vi "Chamber controller Dec 14 2017.vi"() -> ()   [LabVIEW 2014]
doc: "This template is for the Queued Message Handler design pattern.\n\nThe Event Handling Loop generates messages based on user interface actions.\n\nThe Message Handling Loop processes messages generated by the Event Handling Loop, or by other messages. The messages are string values, so new messages can be added easily to the Message Cases case structure in the Message Handling Loop. Each message cluster can also provide an optional value for Message Data, which is a variant that can be converted to whatever message-specific data is required."
uses:
  <vilib>/Analysis/baseanly.llb/Mean (DBL).vi
  <vilib>/Instr/_visa.llb/VISA Configure Serial Port (Instr).vi
  Environmental Chamber LabVIEW and Instruments/Drivers and Software/Keithley 2100 Series/Public/Configure/Configure 2 Wire Resistance.vi
  <vilib>/Utility/file.llb/Write To Spreadsheet File (string).vi
  <vilib>/Utility/file.llb/Read From Spreadsheet File (string).vi
  Environmental Chamber LabVIEW and Instruments/Drivers and Software/LabVIEW 8.2 Drivers/keithley_24xx/Keithley 24XX/Public/Data/Read (Single Point).vi
  Environmental Chamber LabVIEW and Instruments/Drivers and Software/keithley_6430/Keithley 6430/Public/Data/Read (Single Point).vi
  Environmental Chamber LabVIEW and Instruments/Drivers and Software/keithley_6430/Keithley 6430/Keithley 6430.lvlib
  Environmental Chamber LabVIEW and Instruments/Drivers and Software/Keithley 2100 Series/Keithley 2100 Series.lvlib
  Environmental Chamber LabVIEW and Instruments/Drivers and Software/keithley_24xx/Keithley 24XX/Keithley 24XX.lvlib
  <vilib>/Analysis/NI_AALBase.lvlib
panel:
  in  "K2420 Applied Voltage (V)":dbl=0.05
  in  "SYSTEM CONTROL":T1={"valve % open"=0.0, "Desired pressure"=0.0, "set Vapor sccm"=0.0, "set Gas sccm"=0.0, "Valve mode"=enum."% Open", "Pressure Mode"=enum."Abs. pressure", "analyte partial pressure"=23.8, "Actual"=0.0, "Read pressure (Torr)"=0.0, "Read vapor flow (sccm)"=0.0, "Read gas flow (sccm)"=0.0, "Save now"=FALSE, "Stop after seq."=TRUE, "Turbo pump\nauto on"=TRUE, "Integrate points"=0} caption="Pressure settings" {"Integrate points" min=0 max=100 step=1; "analyte partial pressure" min=0.0 max=100.0 step=5.0; "set Gas sccm" min=0 max=200 step=5; "set Vapor sccm" min=0 max=200 step=5; "Desired pressure" min=0.0 max=760.0 step=5.0; "valve % open" min=0.0 max=100.0 step=5.0 format="%#_2f"}
  in  "SAVE SAMPLE / ANALYTE NAMES":T2={"QCM1"="", "QCM2"="", "QCM3"="", "QCM4"="broken", "QCM5"="NOT WORKING", "QCM6"="", "SRS"="bareAu", "K-2420"="", "K-6430"="", "K-2100"="", "Gas"="NOT WORKING", "Vapor"="H2O", "Notes"=""} caption="Save samplffe names"
  in  "Clear all charts":bool
  out "K-6430":dbl(graph)
  out "K-2420":dbl(graph)
  out "File":path caption="DATA FILE"
  in  "Stop":bool
  out "QCM plot":T3(graph)
  out "K-2100":dbl(graph)
  out "State date/time":string caption="Program start time"
  out "J-KEM temp":dbl(graph)
  out "saving data?":bool
  out "pressure chart":dbl(graph)
  out "arduino qcm stack plot":T4(graph)
  in  "SEQUENCE":T5 {"preview" items=["pressure", "gas flow", "vapor flow", "bias"]}
  # "100"
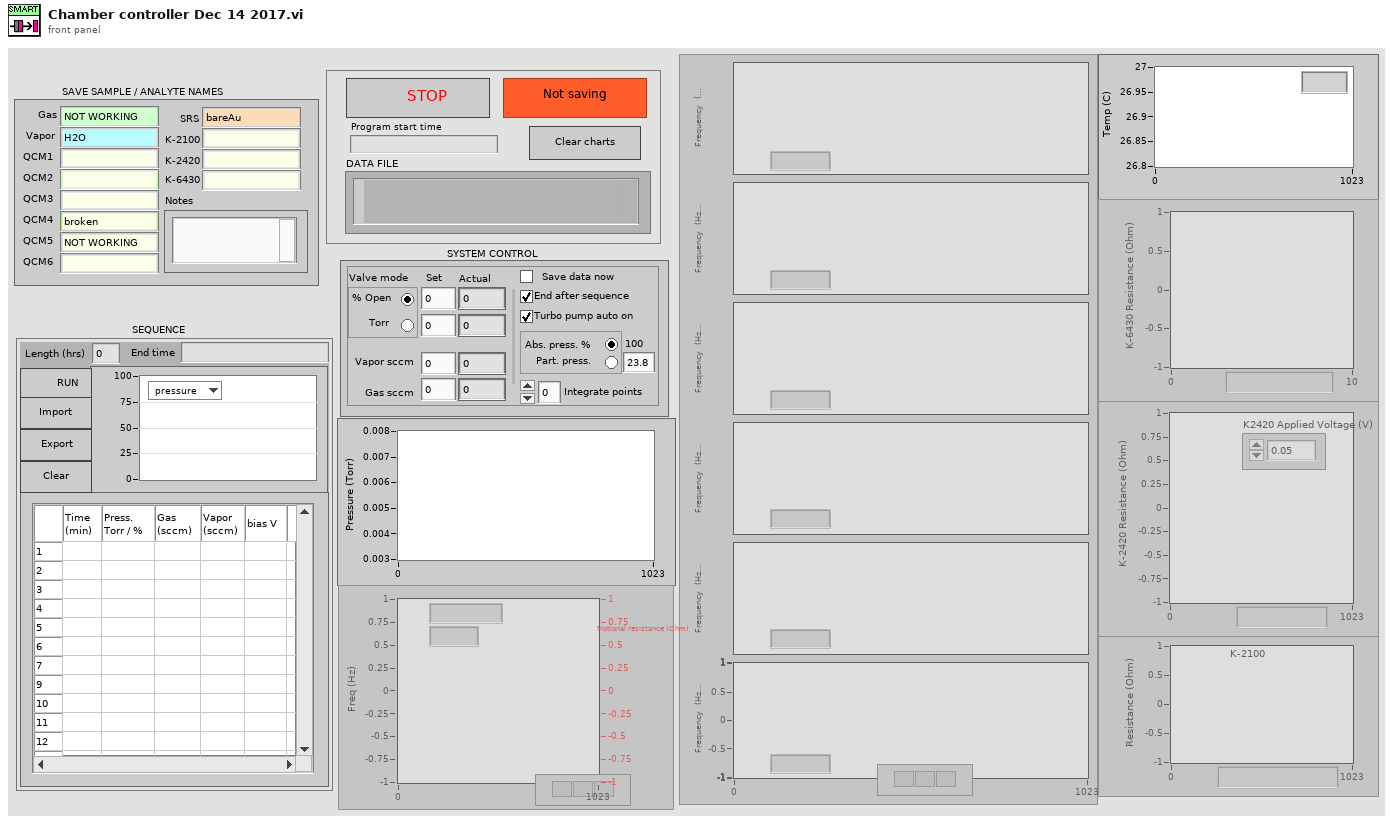
[diagram p1: front panel]
types:
  T1 = cluster{"valve % open":dbl, "Desired pressure":dbl, "set Vapor sccm":sgl, "set Gas sccm":sgl, "Valve mode":enum32{"% Open", "Torr "}, "Pressure Mode":enum32{"Abs. pressure", " Part. pressure"}, "analyte partial pressure":dbl, "Actual":dbl, "Read pressure (Torr)":dbl, "Read vapor flow (sccm)":dbl, "Read gas flow (sccm)":dbl, "Save now":bool, "Stop after seq.":bool, "Turbo pump\nauto on":bool, "Integrate points":i32}
  T2 = cluster{"QCM1":string, "QCM2":string, "QCM3":string, "QCM4":string, "QCM5":string, "QCM6":string, "SRS":string, "K-2420":string, "K-6430":string, "K-2100":string, "Gas":string, "Vapor":string, "Notes":string}
  T3 = cluster{"Frequency out":dbl, "Resistance out":dbl}
  T4 = cluster{"[0]":dbl, "[1]":dbl, "[2]":dbl, "[3]":dbl, "[4]":dbl, "[5]":dbl}
  T5 = cluster{"Run Sequence":bool, "User-defined\nsequence":string[][], "preview":u16, "Sequence\npreview":cluster{dbl[], dbl[]}[], "Save sequence":bool, "Clear sequence":bool, "Import sequence file":bool, "Length (hrs)":dbl, "End time":string}
  T6 = cluster{"Keithley 6430":bool, "J-KEM":bool, "Keithley 2420":bool, "Keithley 2100":bool, "SRS QCM":bool, "Pressure control":bool, "Arduino":bool}
  T7 = cluster{"Arduino 1":refnum<visa-resource-name>, "Arduino 2":refnum<visa-resource-name>, "Arduino 3":refnum<visa-resource-name>, "Arduino 4":refnum<visa-resource-name>, "Arduino 5":refnum<visa-resource-name>, "Arduino 6":refnum<visa-resource-name>}
  T8 = enum8{"Enabled", "Disabled", "Disabled and Grayed Out"}
  T9 = enum16{"open", "open or create", "create or replace", "create", "open (read only)"}
  T10 = cluster{"[0]":dbl, "[1]":dbl, "[2]":dbl, "[3]":dbl, "[4]":dbl, "[5]":dbl}[]
  T11 = cluster{"Frequency out":dbl, "Resistance out":dbl}[]
  T12 = cluster{"VISA resource name":refnum<visa-resource-name>, "error out":errorcluster, bool}
  T13 = cluster{"VISA resource name out":refnum<visa-resource-name>, "error out":errorcluster, bool}
  T14 = cluster{bool, "task out":refnum<k21>, "error out":errorcluster, "task out":refnum<k21>, "error out":errorcluster, "turbo pump":refnum<visa-resource-name>, "error out":errorcluster}
  T15 = cluster{bool, "task out":refnum<k21>, "error out":errorcluster, "task out":refnum<k21>, "error out":errorcluster, "VISA resource name out":refnum<visa-resource-name>, "error out":errorcluster}
  T16 = cluster{bool, "VISA resource name":refnum<visa-resource-name>, "error out":errorcluster}
  T17 = cluster{bool, "VISA resource name out":refnum<visa-resource-name>, "error out":errorcluster}
  T18 = cluster{bool, "VISA in":refnum<visa-resource-name>, "error out":errorcluster}
  T19 = cluster{bool, "VISA out":refnum<visa-resource-name>, "error out":errorcluster}
  T20 = cluster{"Arduino address":refnum<visa-resource-name>, "error in (no error)":errorcluster, "Arduino address 2":refnum<visa-resource-name>, "error in (no error) 2":errorcluster, "Arduino address 3":refnum<visa-resource-name>, "error in (no error) 3":errorcluster, "Arduino address 4":refnum<visa-resource-name>, "error in (no error) 4":errorcluster, "Arduino address 5":refnum<visa-resource-name>, "error in (no error) 5":errorcluster, "Arduino address 6":refnum<visa-resource-name>, "error in (no error) 6":errorcluster, "arduinos on?":bool}
  T21 = cluster{"valve % open":dbl, "Desired pressure":dbl, "set Vapor sccm":sgl, "set Gas sccm":sgl, "Valve mode":enum32{"% Open", "Torr "}, "Pressure Mode":enum32{"Abs. pressure", " Part. pressure"}, "analyte partial pressure":dbl}
  T22 = cluster{"Boolean":bool, "VISA resource name out":refnum<visa-resource-name>, "error out":errorcluster}
  T23 = cluster{"Boolean":bool, "VISA out":refnum<visa-resource-name>, "error out":errorcluster}
  T24 = cluster{"Boolean":bool, "Arduino address":refnum<visa-resource-name>, "error in (no error)":errorcluster, "Arduino address 2":refnum<visa-resource-name>, "error in (no error) 2":errorcluster, "Arduino address 3":refnum<visa-resource-name>, "error in (no error) 3":errorcluster, "Arduino address 4":refnum<visa-resource-name>, "error in (no error) 4":errorcluster, "Arduino address 5":refnum<visa-resource-name>, "error in (no error) 5":errorcluster, "Arduino address 6":refnum<visa-resource-name>, "error in (no error) 6":errorcluster}
  T25 = cluster{"arduino addresses out":cluster{"Boolean":bool, "Arduino address":refnum<visa-resource-name>, "error in (no error)":errorcluster, "Arduino address 2":refnum<visa-resource-name>, "error in (no error) 2":errorcluster, "Arduino address 3":refnum<visa-resource-name>, "error in (no error) 3":errorcluster, "Arduino address 4":refnum<visa-resource-name>, "error in (no error) 4":errorcluster, "Arduino address 5":refnum<visa-resource-name>, "error in (no error) 5":errorcluster, "Arduino address 6":refnum<visa-resource-name>, "error in (no error) 6":errorcluster}, cluster{bool, "VISA resource name out":refnum<visa-resource-name>, "error out":errorcluster}, "Address out":cluster{"Boolean":bool, "VISA resource name out":refnum<visa-resource-name>, "error out":errorcluster}, cluster{bool, "VISA resource name out":refnum<visa-resource-name>, "error out":errorcluster}, cluster{bool, "VISA resource name out":refnum<visa-resource-name>, "error out":errorcluster}, "SRS address out":cluster{"Boolean":bool, "VISA out":refnum<visa-resource-name>, "error out":errorcluster}}
  T26 = cluster{"User-defined\nsequence":string[][], "Present (s)":dbl, "current  step # in":i32, "sequence end time in":timestamp}
  T27 = cluster{"current  step # in":i32, "sequence end time in":timestamp, "Boolean":bool}
  T28 = cluster{"press/RH/gas/vapor":cluster{"pressure":string, "RH":string, "gas flow":string, "vapor flow":string}, "Cluster":cluster{"Valve position (%)":dbl, "read pressure":dbl, "read vapor flow":dbl, "read gas flow":dbl}}
  T29 = cluster{"Boolean":bool, "task out":refnum<k21>, "error out":errorcluster, "task out":refnum<k21>, "error out":errorcluster, "VISA resource name out":refnum<visa-resource-name>, "error out":errorcluster}
  T30 = cluster{"pressure":string, "RH":string, "gas flow":string, "vapor flow":string}
  T31 = cluster{"Valve position (%)":dbl, "read pressure":dbl, "read vapor flow":dbl, "read gas flow":dbl}
  T32 = cluster{"[0]":string, "[1]":string, "[2]":string, "[3]":string, "[4]":string, "[5]":string}
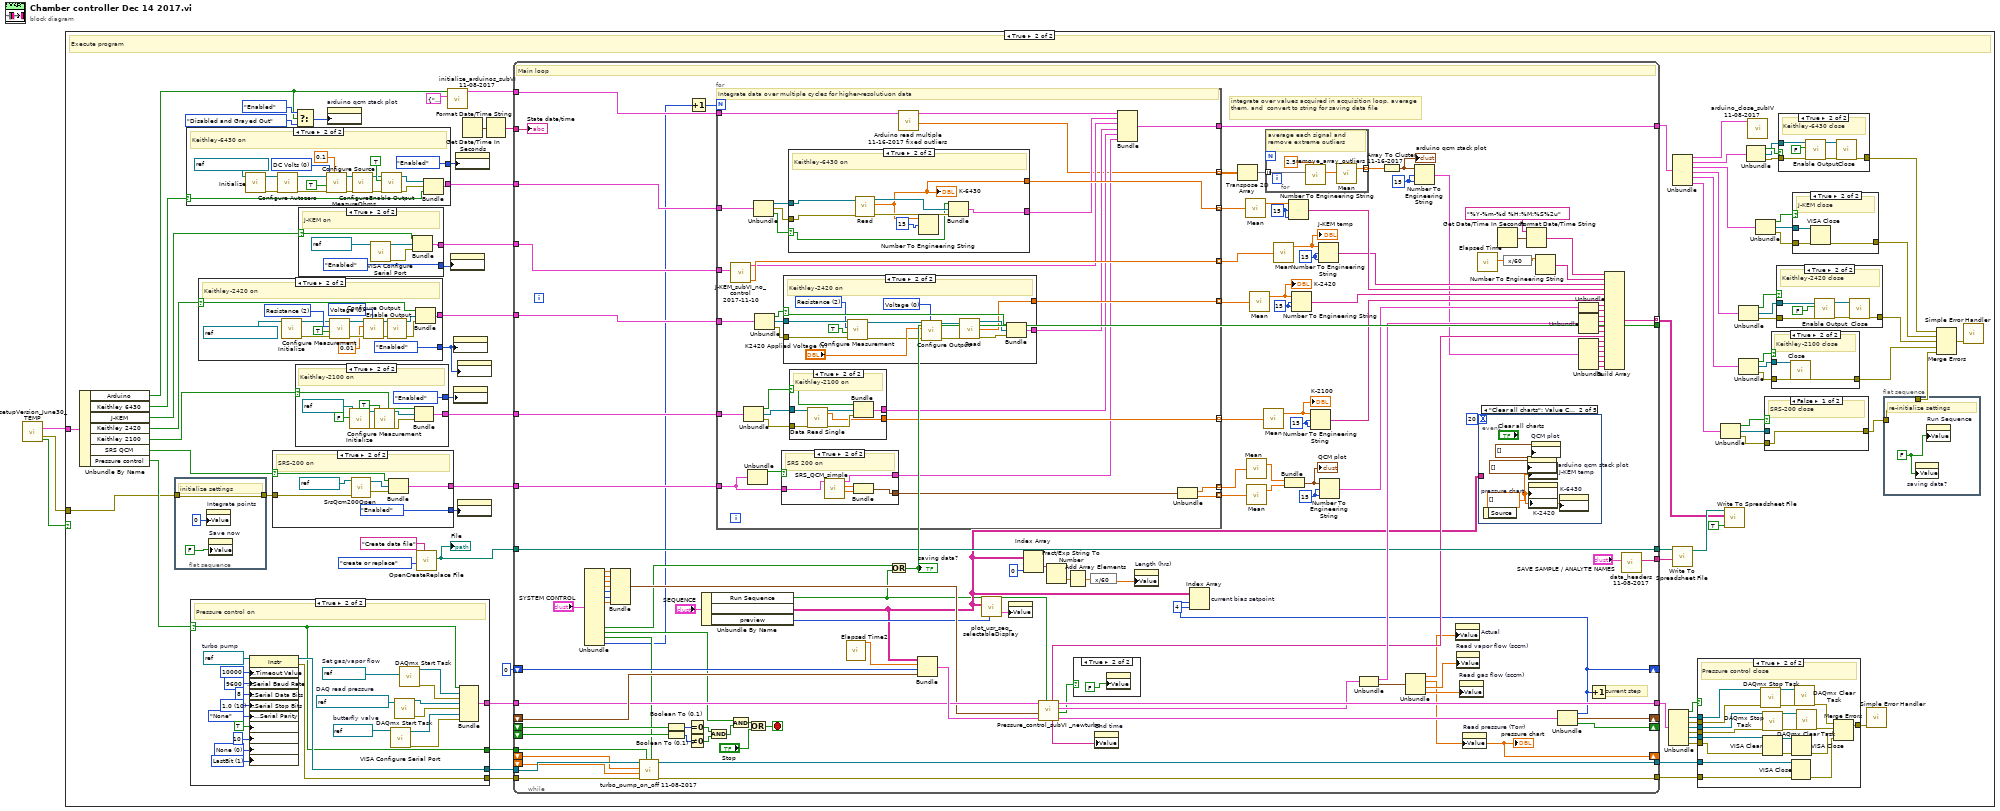
[diagram p0: block diagram]
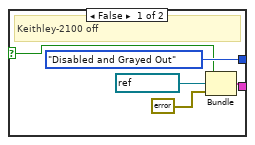
[diagram p4: hidden frame]
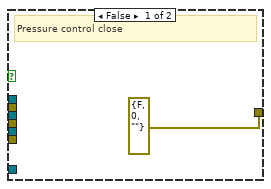
[diagram p5: hidden frame]
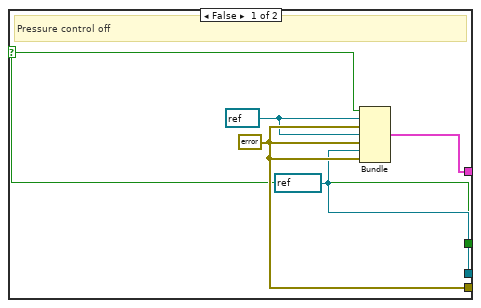
[diagram p6: hidden frame]
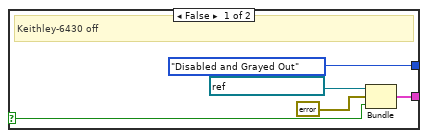
[diagram p8: hidden frame]
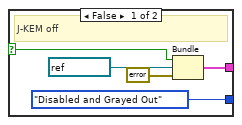
[diagram p10: hidden frame]
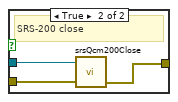
[diagram p11: hidden frame]
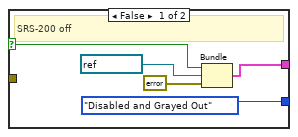
[diagram p12: hidden frame]
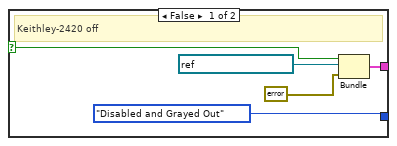
[diagram p14: hidden frame]
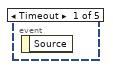
[diagram p15: hidden frame]
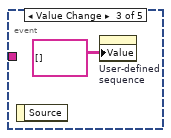
[diagram p16: hidden frame]
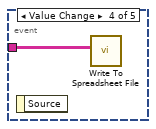
[diagram p17: hidden frame]
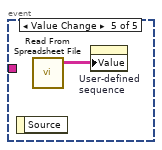
[diagram p18: hidden frame]
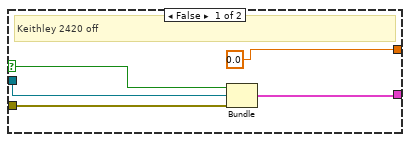
[diagram p19: hidden frame]
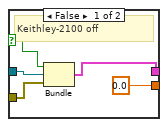
[diagram p20: hidden frame]
diagram:
  n1 = call "setupVersion_June30_TEMP.vi"() -> ("Instruments on/off"=w1:T6, "error IO"=w2:errorcluster, "OK"=w3:bool)  [unwired: 13 in]
  n2 = case shown="True" w3 {
    tunnel: w2 -> [_ w41]
    tunnel: w1 -> [_ w48]
    frame False {
      # "Cancel program"
    }
    frame True {
      # "Execute program"
      n3 = Unbundle By Name(w48) -> ("Arduino"=w19:bool, "Keithley 6430"=w47:bool, "J-KEM"=w46:bool, "Keithley 2420"=w45:bool, "Keithley 2100"=w44:bool, "SRS QCM"=w43:bool, "Pressure control"=w42:bool)
      n4 = flat-sequence {
        tunnel: [w86] -> w40
        tunnel: w41 -> [w86]
        frame #0 {
          # "initialize settings"
          n5 = property on="Integrate points" class="DigNum (strict)"("Value"=0) -> ()  [unwired: 2 in, 2 out]
          n6 = property on="Save now" class="Bool (strict)"("Value"=FALSE) -> ()  [unwired: 2 in, 2 out]
        }
      }
      n7 = case shown="True" w47 {
        selector: w47 -> [w164 w184]
        tunnel: [T8."Disabled and Grayed Out" ("Disabled") T8."Enabled" ("Disabled")] -> w26
        tunnel: [w163 w183] -> w24
        frame False {
          # "Keithley-6430 off"
          n8 = Bundle("VISA resource name"=refnum<visa-resource-name> "GPIB0::29::INSTR", "error out"=errorcluster {"status"=FALSE, "code"=0, "source"=""}, w164) -> (w163:T12)  [unwired: 1 in]
        }
        frame True {
          w171 = u16 0 items=["DC Volts", "DC Current"] ("Source Function (0: DC Volts)")
          # "Keithley-6430 on"
          n9 = call "Initialize.vi"("VISA resource name"=refnum<visa-resource-name> "GPIB2::19::INSTR") -> ("error out"=w177:errorcluster, "VISA resource name out"=w178:refnum<visa-resource-name>)  [unwired: 4 in, 5 out]
          n10 = call "Configure Autozero.vi"("error in (no error)"=w177, "VISA resource name"=w178) -> ("error out"=w174:errorcluster, "VISA resource name out"=w176:refnum<visa-resource-name>)  [unwired: 8 in]
          n11 = call "Configure Source.vi"("V-Source Level [V]"=0.1, "error in (no error)"=w174, "Auto Range (T:Enable)"=TRUE, "Source Function (0: DC Volts)"=w171, "VISA resource name"=w176) -> ("error out"=w173:errorcluster, "VISA resource name out"=w175:refnum<visa-resource-name>)  [unwired: 5 in]
          n12 = call "Configure MeasureOhms.vi"("error in (no error)"=w173, "VISA resource name"=w175) -> ("error out"=w182:errorcluster, "VISA resource name out"=w180:refnum<visa-resource-name>)  [unwired: 4 in, 4 out]
          n13 = call "Enable Output.vi"("error in (no error)"=w182, "Enable Output (F:Off)"=TRUE ("Output (F:Off)"), "VISA resource name"=w180) -> ("error out"=w169:errorcluster, "VISA resource name out"=w170:refnum<visa-resource-name>)  [unwired: 7 out]
          n14 = Bundle("VISA resource name out"=w170, "error out"=w169, w184) -> (w183:T13)  [unwired: 1 in]
        }
      }
      n15 = case shown="True" w42 {
        selector: w42 -> [w128 w134]
        tunnel: [w132 w135] -> w39
        tunnel: [w131 w133] -> w31
        tunnel: [w129 w136] -> w32
        tunnel: [w128 w134] -> w30
        frame False {
          w129 = refnum<visa-resource-name> refnum ("turbo pump")
          w130 = refnum<k21> refnum ("task out")
          w131 = errorcluster {"status"=FALSE, "code"=0, "source"=""} ("error out")
          # "Pressure control off"
          n16 = Bundle(w128, "task out"=w130, "error out"=w131, "task out"=w130, "error out"=w131, "turbo pump"=w129, "error out"=w131) -> (w132:T14)  [unwired: 1 in]
        }
        frame True {
          w140 = u16 1 items=["None", "LastBit", "TermChar"] ("Serial Settings:Serial End Mode for Reads")
          w138 = u16 0 items=["None", "XON/XOFF", "RTS/CTS", "XON/XOFF & RTS/CTS", "DTR/DSR", "XON/XOFF & DTR/DSR"] ("flow control (0:none)")
          w141 = u16 10 items=["1.0"=10, "1.5"=15, "2.0"=20] ("stop bits (10: 1 bit)")
          w137 = refnum<visa-resource-name> "COM7"  # turbo pump
          w153 = refnum<visa-resource-name> "COM5"  # butterfly valve
          w154 = refnum<k21> "Setflow"  # Set gas/vapor flow
          w155 = refnum<k21> "AllDaqReadings"  # DAQ read pressure
          # "Pressure control on"
          n17 = property class="Instr"(reference=w137, "General Settings:Timeout Value"=u32 10000 ("timeout (10sec)"), "Serial Settings:Serial Baud Rate"=u32 9600 ("baud rate (9600)"), "Serial Settings:Serial Data Bits"=u16 8 ("data bits (8)"), "Serial Settings:Serial Stop Bits"=w141, "Serial Settings:Serial Parity"=enum16{"None", "Odd", "Even", "Mark", "Space"}."None" ("parity (0:none)"), "Message Based Settings:Termination Character Enable"=TRUE ("Enable Termination\nChar (T)"), "Message Based Settings:Termination Character"=u8 10 ("termination char\n(0xA = '\\n' = LF)"), "Serial Settings:Serial Flow Control"=w138, "Serial Settings:Serial End Mode for Reads"=w140) -> (reference out=w136:refnum<visa-resource-name>, error out=w133:errorcluster)  [unwired: 1 in]
          n18 = call-poly "VISA Configure Serial Port"("VISA resource name"=w153) -> ("VISA resource name out"=w148:refnum<visa-resource-name>, "error out"=w147:errorcluster)  [unwired: 13 in]
          n19 = call <vilib>:"DAQmx Start Task.vi"("task/channels in"=w155) -> ("task out"=w150:refnum<k21>, "error out"=w149:errorcluster)  [unwired: 13 in]
          n20 = call <vilib>:"DAQmx Start Task.vi"("task/channels in"=w154) -> ("task out"=w152:refnum<k21>, "error out"=w151:errorcluster)  [unwired: 13 in]
          n21 = Bundle(w134, "task out"=w152, "error out"=w151, "task out"=w150, "error out"=w149, "VISA resource name out"=w148, "error out"=w147) -> (w135:T15)  [unwired: 1 in]
        }
      }
      n22 = case shown="True" w45 {
        selector: w45 -> [w227 w232]
        tunnel: [T8."Disabled and Grayed Out" ("Disabled") T8."Enabled" ("Disabled")] -> w4
        tunnel: [w225 w229] -> w23
        frame False {
          # "Keithley-2420 off"
          n23 = Bundle(w227, "VISA resource name"=refnum<visa-resource-name> "GPIB1::24::INSTR", "error out"=errorcluster {"status"=FALSE, "code"=0, "source"=""}) -> (w225:T16)  [unwired: 1 in]
        }
        frame True {
          w238 = u16 0 items=["Voltage", "Current"] ("Source Mode  (0: Voltage)")
          w243 = u16 2 items=["Volts", "Current", "Resistance"] ("Function (0: Volts)")
          # "Keithley-2420 on"
          n24 = call "Initialize.vi"("VISA resource name"=refnum<visa-resource-name> "GPIB1::24::INSTR") -> ("error out"=w233:errorcluster, "VISA resource name out"=w234:refnum<visa-resource-name>)  [unwired: 9 in]
          n25 = call "Configure Measurement.vi"("error in (no error)"=w233, "Enable Auto Range (T:Enable)"=TRUE, "Function (0: Volts)"=w243, "VISA resource name"=w234) -> ("error out"=w242:errorcluster, "VISA resource name out"=w241:refnum<visa-resource-name>)  [unwired: 6 in]
          n26 = call "Configure Output.vi"("Source Mode  (0: Voltage)"=w238, "error in (no error)"=w242, "Output Level (0)"=0.01 ("K2420 Applied Voltage (V) 2"), "VISA resource name"=w241) -> ("error out"=w240:errorcluster, "VISA resource name out"=w239:refnum<visa-resource-name>)  [unwired: 6 in]
          n27 = call "Enable Output.vi"("error in (no error)"=w240, "VISA resource name"=w239) -> ("error out"=w230:errorcluster, "VISA resource name out"=w231:refnum<visa-resource-name>)  [unwired: 8 in]
          n28 = Bundle(w232, "VISA resource name out"=w231, "error out"=w230) -> (w229:T17)  [unwired: 1 in]
        }
      }
      n29 = case shown="True" w43 {
        selector: w43 -> [w206 w212]
        tunnel: w40 -> [_ w215]
        tunnel: [T8."Disabled and Grayed Out" ("Disabled") T8."Enabled" ("Disabled")] -> w63
        tunnel: [w205 w211] -> w21
        frame False {
          # "SRS-200 off"
          n30 = Bundle(w206, "VISA in"=refnum<visa-resource-name> "COM6", "error out"=errorcluster {"status"=FALSE, "code"=0, "source"=""}) -> (w205:T18)  [unwired: 1 in]
        }
        frame True {
          # "SRS-200 on"
          n31 = call "SrsQcm200Open.vi"("error in"=w215, "VISA in"=refnum<visa-resource-name> "COM6") -> ("error out"=w210:errorcluster, "VISA out"=w213:refnum<visa-resource-name>)  [unwired: 3 in]
          n32 = Bundle(w212, "VISA out"=w213, "error out"=w210) -> (w211:T19)  [unwired: 1 in]
        }
      }
      n33 = Select(t=T8."Enabled" ("Disabled"), s=w19, f=T8."Disabled and Grayed Out" ("Disabled")) -> (s? t:f=w27:T8)
      n34 = case shown="True" w44 {
        selector: w44 -> [w96 w100]
        tunnel: [T8."Disabled and Grayed Out" ("Disabled") T8."Enabled" ("Disabled")] -> w58
        tunnel: [w93 w101] -> w22
        frame False {
          # "Keithley-2100 off"
          n35 = Bundle(w96, "VISA resource name out"=refnum<visa-resource-name> "K-2100", "error out"=errorcluster {"status"=FALSE, "code"=0, "source"=""}) -> (w93:T17)  [unwired: 1 in]
        }
        frame True {
          # "Keithley-2100 on"
          n36 = call "Initialize.vi"("VISA resource name"=refnum<visa-resource-name> "K-2100", "Reset? (T: Reset)"=FALSE) -> ("VISA resource name out"=w105:refnum<visa-resource-name>, "error out"=w104:errorcluster)  [unwired: 16 in]
          n37 = call-poly "Configure Measurement.vi"("VISA resource name"=w105, "error in (no error)"=w104, "Auto Range? (T: Auto)"=TRUE) -> ("VISA resource name out"=w99:refnum<visa-resource-name>, "error out"=w98:errorcluster)  [unwired: 15 in]
          n38 = Bundle(w100, "VISA resource name out"=w99, "error out"=w98) -> (w101:T17)  [unwired: 1 in]
        }
      }
      n39 = case shown="True" w46 {
        selector: w46 -> [w191 w197]
        tunnel: [w192 w198] -> w76
        tunnel: [T8."Disabled and Grayed Out" ("Disabled") T8."Enabled" ("Disabled")] -> w25
        frame False {
          # "J-KEM off"
          n40 = Bundle(w191, "VISA resource name"=refnum<visa-resource-name> "COM3", "error out"=errorcluster {"status"=FALSE, "code"=0, "source"=""}) -> (w192:T16)  [unwired: 1 in]
        }
        frame True {
          # "J-KEM on"
          n41 = call-poly "VISA Configure Serial Port"("VISA resource name"=refnum<visa-resource-name> "COM3") -> ("VISA resource name out"=w199:refnum<visa-resource-name>, "error out"=w196:errorcluster)  [unwired: 13 in]
          n42 = Bundle(w197, "VISA resource name out"=w199, "error out"=w196) -> (w198:T17)  [unwired: 1 in]
        }
      }
      n43 = property on="arduino qcm stack plot" class="WFChart (strict)"("DisabledEnum"=w27) -> ()  [unwired: 2 in, 2 out]
      n44 = call "OpenCreateReplace File.vi"("prompt"="Create data file", "function (open:0)"=T9."create or replace") -> ("new file path"=w20:path)  [unwired: 6 in, 3 out]
      "File" <- w20
      n45 = call "initialize_arduinos_subVI 11-08-2017.vi"("arduino 1-6 addresses"=T7 {"Arduino 1"="COM25", "Arduino 2"="COM48", "Arduino 3"="COM21", "Arduino 4"="COM22", "Arduino 5"="COM23", "Arduino 6"="COM24"} ("Arduino COMs"), "arduinos on?"=w19) -> ("arduino addresses out"=w61:T20)  [unwired: 9 in]
      n46 = property on="J-KEM temp" class="WFChart (strict)"("DisabledEnum"=w25) -> ()  [unwired: 2 in, 2 out]
      n47 = property on="K-2420" class="WFChart (strict)"("DisabledEnum"=w4) -> ()  [unwired: 2 in, 2 out]
      n48 = property on="K-2100" class="WFChart (strict)"("DisabledEnum"=w58) -> ()  [unwired: 2 in, 2 out]
      n49 = property on="K-6430" class="WFChart (strict)"("DisabledEnum"=w26) -> ()  [unwired: 2 in, 2 out]
      n50 = property on="K2420 Applied Voltage (V)" class="DigNum (strict)"("DisabledEnum"=w4) -> ()  [unwired: 2 in, 2 out]
      n51 = property on="QCM plot" class="WFChart (strict)"("DisabledEnum"=w63) -> ()  [unwired: 2 in, 2 out]
      n52 = Get Date/Time In Seconds() -> (seconds since 1Jan1904=w5:timestamp)
      n53 = Format Date/Time String(seconds (now)=w5) -> (date/time string=w57:string)  [unwired: 2 in]
      n54 = while {
        tunnel: [w364] -> w62 mode=indexing if=w351
        tunnel: w76 -> [w366]
        tunnel: [w334] -> w68
        tunnel: w20 -> [w334]
        tunnel: [w351] -> _
        tunnel: w61 -> [w311]
        tunnel: [w323] -> w60
        tunnel: w57 -> [w346]
        tunnel: w39 -> [w332]
        shift-right: [w307] -> _
        shift-left: 0 ("1st step") -> [w338]
        shift-right: [w343] -> _
        shift-left: _ -> [w341]
        shift-right: [w342] -> _
        shift-left: _ -> [w340]
        shift-left: _ -> [w339]
        tunnel: [w337] -> w53
        tunnel: w32 -> [w331]
        tunnel: w31 -> [w330]
        tunnel: w30 -> [w310]
        tunnel: [w328] -> w29
        tunnel: [w329] -> w28
        tunnel: w24 -> [w316]
        tunnel: w23 -> [w315]
        tunnel: w22 -> [w314]
        tunnel: w21 -> [w313]
        shift-right: [w246] -> _
        shift-left: _ -> [w309]
        shift-left: _ -> [w308]
        tunnel: [w281] -> w12
        stop <- w353 stop-if-true
        w273 = i16 15 ("width (-)")
        w274 = i16 15 ("width (-)")
        w275 = i16 15 ("width (-)")
        w276 = i16 15 ("width (-)")
        w277 = i16 15 ("width (-)")
        w278 = i16 15 ("width (-)")
        # "current step"
        # "integrate over values acquired in acquisition loop, average them, and  convert to string for saving data file"
        # "Main loop"
        n55 = Unbundle("SYSTEM CONTROL") -> ("valve % open"=w266:dbl, "Desired pressure"=w265:dbl, "set Vapor sccm"=w264:sgl, "set Gas sccm"=w263:sgl, "Valve mode"=w262:enum32{"% Open", "Torr "}, "Pressure Mode"=w261:enum32{"Abs. pressure", " Part. pressure"}, "analyte partial pressure"=w260:dbl, "Save now"=w251:bool, "Stop after seq."=w250:bool, "Turbo pump\nauto on"=w249:bool, "Integrate points"=w248:i32)  [unwired: 4 out]
        n56 = Bundle("valve % open"=w266, "Desired pressure"=w265, "set Vapor sccm"=w264, "set Gas sccm"=w263, "Valve mode"=w262, "Pressure Mode"=w261, "analyte partial pressure"=w260) -> (w267:T21)  [unwired: 1 in]
        n57 = call "turbo_pump_on_off 11-08-2017.vi"("Turbo pump\nauto on"=w249, "pressure control on?"=w310, "error in (no error)"=w330, "read pressure"=w308, "read pressure 2"=w309, "VISA Refnum in"=w331) -> ("error out"=w329:errorcluster, "VISA Refnum out"=w328:refnum<visa-resource-name>)  [unwired: 4 in]
        n58 = Boolean To (0,1)(Boolean=w340) -> (0, 1=w357:i16)
        n59 = Boolean To (0,1)(Boolean=w339) -> (0, 1=w356:i16)
        n60 = Equal To 0?(x=w357) -> (x = 0?=w354:bool)
        n61 = Not Equal To 0?(x=w356) -> (x != 0?=w355:bool)
        n62 = Increment(x=w248) -> (x+1=w280:i32)
        n63 = Unbundle By Name("SEQUENCE") -> ("Run Sequence"=w253:bool, "User-defined\nsequence"=w257:string[][], "preview"=w258:u16)
        n64 = And(x=w354, y=w355) -> (x .and. y?=w352:bool)
        n65 = for {
          N: w280 -> [_]
          tunnel: w316 -> [w407]
          tunnel: w315 -> [w404]
          tunnel: w314 -> [w400]
          tunnel: w313 -> [w381]
          tunnel: w311 -> [w380]
          tunnel: w366 -> [w408]
          tunnel: [w395] -> w302 mode=indexing
          tunnel: [w394] -> w296 mode=indexing
          tunnel: [w393] -> w299 mode=indexing
          tunnel: [w392] -> w294 mode=indexing
          tunnel: [w390] -> w292 mode=indexing
          tunnel: [w389] -> w291 mode=indexing
          tunnel: [w379] -> w286 mode=indexing
          tunnel: [w383] -> w281
          # "Integrate data over multiple cycles for higher-resolutiuon data"
          n66 = call "J-KEM_subVI_no_control 2017-11-10.vi"("Address in"=w408) -> ("Temp (C)"=w393:dbl, "Address out"=w387:T22)  [unwired: 9 in]
          n67 = Unbundle(w400) -> (w399:bool, "VISA resource name out"=w398:refnum<visa-resource-name>, "error out"=w397:errorcluster)
          n68 = Unbundle(w381) -> (w382:bool)  [unwired: 2 out]
          n69 = Unbundle(w407) -> ("VISA resource name out"=w406:refnum<visa-resource-name>, "error out"=w396:errorcluster, w405:bool)
          n70 = Unbundle(w404) -> (w403:bool, "VISA resource name out"=w402:refnum<visa-resource-name>, "error out"=w401:errorcluster)
          n71 = case "SRS QCM" shown="True" w382 {
            tunnel: [w454 w460] -> w384
            tunnel: [T3 {"Frequency out"=0.0, "Resistance out"=0.0} ("freq, MR") w457] -> w391
            tunnel: w381 -> [w454 w456]
            frame False {
              # "SRS QCM off"
            }
            frame True {
              # "SRS 200 on"
              n72 = call "SRS_QCM_simple.vi"("SRS address in"=w456) -> ("Resistance out"=w459:dbl, "Frequency out"=w458:dbl, "SRS address out"=w460:T23)  [unwired: 8 in]
              n73 = Bundle("Frequency out"=w458, "Resistance out"=w459) -> (w457:T3)  [unwired: 1 in]
            }
          }
          n74 = case shown="True" w403 {
            selector: w403 -> [w413 w428]
            tunnel: [w410 w427] -> w386
            tunnel: w402 -> [w412 w420]
            tunnel: w401 -> [w411 w418]
            tunnel: [sgl 0.0 ("Resistance") w415] -> w394
            frame False {
              # "Keithley 2420 off"
              n75 = Bundle(w413, "VISA resource name out"=w412, "error out"=w411) -> (w410:T17)  [unwired: 1 in]
            }
            frame True {
              w416 = u16 2 items=["Volts", "Current", "Resistance"] ("Function (0: Volts)")
              w424 = u16 0 items=["Voltage", "Current"] ("Source Mode  (0: Voltage)")
              # "Keithley-2420 on"
              n76 = call "Configure Measurement.vi"("error in (no error)"=w418, "Enable Auto Range (T:Enable)"=TRUE, "Function (0: Volts)"=w416, "VISA resource name"=w420) -> ("error out"=w417:errorcluster, "VISA resource name out"=w419:refnum<visa-resource-name>)  [unwired: 6 in]
              n77 = call "Configure Output.vi"("Source Mode  (0: Voltage)"=w424, "error in (no error)"=w417, "Output Level (0)"="K2420 Applied Voltage (V)", "VISA resource name"=w419) -> ("error out"=w422:errorcluster, "VISA resource name out"=w423:refnum<visa-resource-name>)  [unwired: 6 in]
              n78 = call-poly "Read.vi"("VISA resource name"=w423, "error in (no error)"=w422) -> ("VISA resource name out"=w426:refnum<visa-resource-name>, "Resistance"=w415:sgl, "error out"=w425:errorcluster)  [unwired: 7 in, 4 out]
              n79 = Bundle(w428, "VISA resource name out"=w426, "error out"=w425) -> (w427:T17)  [unwired: 1 in]
            }
          }
          n80 = case "Keithley 6430" shown="True" w405 {
            selector: w405 -> [w445 w448]
            tunnel: w406 -> [w444 w450]
            tunnel: [w443 w447] -> w388
            tunnel: w396 -> [w442 w449]
            tunnel: [0.0 ("K6340 Bias (V)") w446] -> w395
            frame False {
              # "Keithley-6430 off"
              n81 = Bundle(w445, "VISA resource name out"=w444, "error out"=w442) -> (w443:T17)  [unwired: 1 in]
            }
            frame True {
              # "Keithley-6430 on"
              n82 = call-poly "Read.vi"("error in (no error)"=w449, "VISA resource name"=w450) -> ("error out"=w451:errorcluster, "Measurement"=w446:dbl, "VISA resource name out"=w452:refnum<visa-resource-name>)  [unwired: 1 in, 6 out]
              "K-6430" <- w446
              n83 = Number To Engineering String(3:i16 15 ("width (-)"), 4:w446) -> ()  [unwired: 2 in, 1 out]
              n84 = Bundle(w448, "VISA resource name out"=w452, "error out"=w451) -> (w447:T17)  [unwired: 1 in]
            }
          }
          n85 = case shown="True" w399 {
            selector: w399 -> [w433 w438]
            tunnel: w398 -> [w431 w440]
            tunnel: w397 -> [w432 w439]
            tunnel: [w430 w435] -> w385
            tunnel: [0.0 ("Measurement") w434] -> w392
            frame False {
              # "Keithley-2100 off"
              n86 = Bundle(w433, "VISA resource name out"=w431, "error out"=w432) -> (w430:T17)  [unwired: 1 in]
            }
            frame True {
              # "Keithley-2100 on"
              n87 = call "Data Read Single.vi"("VISA resource name"=w440, "error in (no error)"=w439) -> ("VISA resource name out"=w437:refnum<visa-resource-name>, "Measurement"=w434:dbl, "error out"=w436:errorcluster)  [unwired: 15 in]
              n88 = Bundle(w438, "VISA resource name out"=w437, "error out"=w436) -> (w435:T17)  [unwired: 1 in]
            }
          }
          n89 = call "Arduino read multiple 11-16-2017 fixed outliers.vi"("arduino addresses in"=w380) -> ("freq out"=w379:dbl[], "arduino addresses out"=w378:T24)  [unwired: 8 in]
          n90 = Bundle("arduino addresses out"=w378, w388, "Address out"=w387, w386, w385, "SRS address out"=w384) -> (w383:T25)  [unwired: 1 in]
          n91 = Unbundle(w391) -> ("Frequency out"=w390:dbl, "Resistance out"=w389:dbl)
        }
        n92 = And(x=w250, y=w352) -> (x .and. y?=w350:bool)
        n93 = Or(x=w350, y="Stop") -> (x .or. y?=w353:bool)
        n94 = call "Elapsed Time2"() -> ("Present (s)"=w272:dbl)  [unwired: 12 in, 7 out]
        n95 = Or(x=w251, y=w253) -> (x .or. y?=w351:bool)
        "saving data?" <- w351
        n96 = Bundle("User-defined\nsequence"=w257, "Present (s)"=w272, "current  step # in"=w338, "sequence end time in"=w341) -> (w345:T26)  [unwired: 1 in]
        n97 = call "plot_usr_seq_selectableDisplay.vi"("Display"=w258, "User-defined sequence"=w257) -> ("Sequence Preview"=w256:cluster{dbl[], dbl[]}[])  [unwired: 9 in]
        n98 = property on="Sequence\npreview" class="XYGraph (strict)"("Value"=w256) -> ()  [unwired: 2 in, 2 out]
        n99 = Index Array(array=w257, index (col)=0 ("disabled index (col)")) -> (element=w326:string[])  [unwired: 1 in]
        n100 = call "Pressure_control_subVI _newturbo.vi"("Run Sequence"=w253, "user sequence, present (s) in, current step in, seq time in"=w345, "pressure parameters in"=w267, "pressure control on?/daq IDs/errors"=w332) -> ("current step # out, shift register time out, seq button on?"=w344:T27, "sequence over? USE THIS TO REINITIALIZE RUN SEQUENCE BUTTON SO PROGRAM ENDS"=w255:bool, "save press/RH/gasflow/vaporflow - read valve position/pressure/vaporflow/gasflow"=w336:T28, "pressure control on?/daq IDs/errors out"=w337:T29, "sequence end date/time string"=w245:string, "pressure_setpoint"=w333:string)  [unwired: 2 in]
        n101 = Fract/Exp String To Number(string=w326) -> (number=w325:dbl[])  [unwired: 3 in, 1 out]
        n102 = Add Array Elements(numeric array=w325) -> (sum=w312:dbl)
        n103 = case shown="True" w255 {
          frame False {
          }
          frame True {
            n104 = property on="Run Sequence" class="Bool (strict)"("Value"=FALSE ("Run Sequence")) -> ()  [unwired: 2 in, 2 out]
          }
        }
        n105 = expression code="x/60"(w312) -> (w247:dbl)
        n106 = property on="End time" class="Str"("Value"=w245) -> ()  [unwired: 2 in, 2 out]
        n107 = property on="Length (hrs)" class="DigNum (strict)"("Value"=w247) -> ()  [unwired: 2 in, 2 out]
        n108 = Transpose 2D Array(2D array=w286) -> (transposed array=w285:dbl[][])
        n109 = call-poly <vilib>:"Mean.vi"("X"=w302) -> ("mean"=w304:dbl)  [unwired: 1 out]
        n110 = call-poly <vilib>:"Mean.vi"("X"=w292) -> ("mean"=w290:dbl)  [unwired: 1 out]
        n111 = call-poly <vilib>:"Mean.vi"("X"=w291) -> ("mean"=w289:dbl)  [unwired: 1 out]
        n112 = call-poly <vilib>:"Mean.vi"("X"=w296) -> ("mean"=w301:dbl)  [unwired: 1 out]
        "K-2420" <- w301
        n113 = call-poly <vilib>:"Mean.vi"("X"=w294) -> ("mean"=w295:dbl)  [unwired: 1 out]
        "K-2100" <- w295
        n114 = for {
          tunnel: w285 -> [w376] mode=indexing
          tunnel: [w377] -> w284 mode=indexing
          # "average each signal and remove extreme outliers"
          n115 = call "remove_array_outliers 11-16-2017.vi"("n standard devs to filter"=2.5, "input array"=w376) -> ("filtered array out"=w375:dbl[])  [unwired: 9 in]
          n116 = call-poly <vilib>:"Mean.vi"("X"=w375) -> ("mean"=w377:dbl)  [unwired: 1 out]
        }
        n117 = call-poly <vilib>:"Mean.vi"("X"=w299) -> ("mean"=w297:dbl)  [unwired: 1 out]
        "J-KEM temp" <- w297
        n118 = Bundle("mean"=w290, "mean"=w289) -> (w288:cluster{"mean":dbl, "mean":dbl})  [unwired: 1 in]
        "QCM plot" <- w288
        n119 = Number To Engineering String(2:w278, 3:w278, 4:w304) -> (0:w303:string)  [unwired: 1 in]
        n120 = Number To Engineering String(2:w276, 3:w276, 4:w301) -> (0:w300:string)  [unwired: 1 in]
        n121 = Number To Engineering String(2:w275, 3:w275, 4:w295) -> (0:w293:string)  [unwired: 1 in]
        n122 = Number To Engineering String(2:w277, 3:w277, 4:w297) -> (0:w298:string)  [unwired: 1 in]
        n123 = Number To Engineering String(2:w273, 3:w273, 4:w288) -> (0:w287:cluster{"mean":string, "mean":string})  [unwired: 1 in]
        n124 = Unbundle(w336) -> ("press/RH/gas/vapor"=w335:T30, "Cluster"=w271:T31)
        n125 = Array To Cluster(array=w284) -> (cluster=w283:T4)
        "arduino qcm stack plot" <- w283
        n126 = Unbundle(w271) -> ("Valve position (%)"=w270:dbl, "read pressure"=w246:dbl, "read vapor flow"=w269:dbl, "read gas flow"=w268:dbl)
        "pressure chart" <- w246
        n127 = Number To Engineering String(2:w274, 3:w274, 4:w283) -> (0:w282:T32)  [unwired: 1 in]
        n128 = property on="Actual" class="DigNum (strict)"("Value"=w270) -> ()  [unwired: 2 in, 2 out]
        n129 = property on="Read vapor flow (sccm)" class="DigNum (strict)"("Value"=w269) -> ()  [unwired: 2 in, 2 out]
        n130 = property on="Read gas flow (sccm)" class="DigNum (strict)"("Value"=w268) -> ()  [unwired: 2 in, 2 out]
        n131 = property on="Read pressure (Torr)" class="DigNum (strict)"("Value"=w246) -> ()  [unwired: 2 in, 2 out]
        n132 = call "Elapsed Time"() -> ("Elapsed Time (s)"=w305:dbl)  [unwired: 12 in, 7 out]
        n133 = event shown="[1] \"Clear all charts\": Value Change" {
          selector: _ -> [_ _ _ _ _]
          dyn-events: _ -> [_ _ _ _ _]
          timeout: 20 -> [_ _ _ _ _]
          tunnel: w257 -> [_ _ _ w372 _]
          event Timeout {
            n134 = event-data() -> ()  [unwired: 1 in, 1 out]
          }
          event "Clear all charts": Value Change {
            w368 = dbl[] [] ("History Data")
            n135 = event-data() -> ()  [unwired: 1 in, 1 out]
            n136 = property on="arduino qcm stack plot" class="WFChart (strict)"("History Data"=T10 []) -> ()  [unwired: 2 in, 2 out]
            n137 = property on="J-KEM temp" class="WFChart (strict)"("History Data"=w368) -> ()  [unwired: 2 in, 2 out]
            n138 = property on="pressure chart" class="WFChart (strict)"("History Data"=w368) -> ()  [unwired: 2 in, 2 out]
            n139 = property on="K-2420" class="WFChart (strict)"("History Data"=w368) -> ()  [unwired: 2 in, 2 out]
            n140 = property on="QCM plot" class="WFChart (strict)"("History Data"=T11 []) -> ()  [unwired: 2 in, 2 out]
            n141 = property on="K-6430" class="WFChart (strict)"("History Data"=w368) -> ()  [unwired: 2 in, 2 out]
          }
          event "SEQUENCE.Clear sequence": Value Change {
            n142 = event-data() -> ()  [unwired: 1 in, 1 out]
            n143 = property on="User-defined\nsequence" class="Tbl (strict)"("Value"=string[][] []) -> ()  [unwired: 2 in, 2 out]
          }
          event "SEQUENCE.Save sequence": Value Change {
            n144 = event-data() -> ()  [unwired: 1 in, 1 out]
            n145 = call-poly <vilib>:"Write To Spreadsheet File.vi"("2D data"=w372) -> ()  [unwired: 7 in, 1 out]
          }
          event "SEQUENCE.Import sequence file": Value Change {
            n146 = event-data() -> ()  [unwired: 1 in, 1 out]
            n147 = call-poly <vilib>:"Read From Spreadsheet File.vi"() -> ("all rows"=w373:string[][])  [unwired: 7 in, 4 out]
            n148 = property on="User-defined\nsequence" class="Tbl (strict)"("Value"=w373) -> ()  [unwired: 2 in, 2 out]
          }
        }
        n149 = Get Date/Time In Seconds() -> (seconds since 1Jan1904=w367:timestamp)
        n150 = expression code="x/60"(w305) -> (w306:dbl)
        n151 = Format Date/Time String(time format string (%c)="%Y-%m-%d %H:%M:%S%2u", seconds (now)=w367) -> (date/time string=w362:string)  [unwired: 1 in]
        n152 = Number To Engineering String ("elapsed time (min)")(4:w306) -> (0:w347:string)  [unwired: 3 in]
        n153 = Unbundle(w344) -> ("current  step # in"=w307:i32, "sequence end time in"=w343:timestamp, "Boolean"=w342:bool)
        n154 = Index Array "current bias setpoint"(array=w257, index (row)=w307, index (col)=4 ("disabled index (col)")) -> ()  [unwired: 1 out]
        n155 = Unbundle(w287) -> ("mean"=w348:string, "mean"=w363:string)
        n156 = Unbundle(w335) -> ("pressure"=w361:string, "RH"=w360:string, "gas flow"=w359:string, "vapor flow"=w358:string)
        n157 = Unbundle(w282) -> ("[0]"=w322:string, "[1]"=w321:string, "[2]"=w320:string, "[3]"=w319:string, "[4]"=w318:string, "[5]"=w317:string)
        n158 = Increment(x=w307) -> ()  [unwired: 1 out]
        n159 = Build Array(w362, w347, w298, w303, w300, w293, w348, w363, w361, w360, w359, w358, w333, w322, w321, w320, w319, w318, w317) -> (w364:string[])
        n160 = call "data_headers 11-08-2017.vi"("Sample names"="SAVE SAMPLE / ANALYTE NAMES") -> ("data headers"=w323:string[])  [unwired: 10 in]
        "State date/time" <- w346
      }
      n161 = Unbundle(w53) -> ("Boolean"=w52:bool, "task out"=w38:refnum<k21>, "error out"=w37:errorcluster, "task out"=w36:refnum<k21>, "error out"=w35:errorcluster, "VISA resource name out"=w34:refnum<visa-resource-name>, "error out"=w33:errorcluster)
      n162 = Unbundle(w12) -> ("arduino addresses out"=w11:T24, w10:T17, "Address out"=w9:T22, w8:T17, w7:T17, "SRS address out"=w6:T23)
      n163 = call-poly <vilib>:"Write To Spreadsheet File.vi"("1D data"=w60, "file path (dialog if empty)"=w68) -> ("new file path (Not A Path if cancelled)"=w71:path)  [unwired: 6 in]
      n164 = case shown="True" w52 {
        tunnel: [errorcluster {"status"=FALSE, "code"=0, "source"=""} ("error out") w119] -> w56
        tunnel: w38 -> [_ w118]
        tunnel: w37 -> [_ w117]
        tunnel: w36 -> [_ w116]
        tunnel: w35 -> [_ w113]
        tunnel: w34 -> [_ w114]
        tunnel: w33 -> [_ w115]
        tunnel: w29 -> [_ w110]
        tunnel: w28 -> [_ w109]
        frame False {
          # "Pressure control close"
        }
        frame True {
          # "Pressure control close"
          n165 = call <vilib>:"DAQmx Stop Task.vi"("task/channels in"=w118, "error in"=w117) -> ("task out"=w125:refnum<k21>, "error out"=w124:errorcluster)  [unwired: 12 in]
          n166 = call <vilib>:"DAQmx Stop Task.vi"("task/channels in"=w116, "error in"=w113) -> ("task out"=w126:refnum<k21>, "error out"=w127:errorcluster)  [unwired: 12 in]
          n167 = VISA Clear(VISA resource name=w114, error in (no error)=w115) -> (VISA resource name out=w123:refnum<visa-resource-name>, error out=w122:errorcluster)
          n168 = VISA Close(VISA resource name=w110, error in (no error)=w109) -> (error out=w111:errorcluster)
          n169 = VISA Close(VISA resource name=w123, error in (no error)=w122) -> (error out=w112:errorcluster)
          n170 = call <vilib>:"DAQmx Clear Task.vi"("task in"=w125, "error in"=w124) -> ("error out"=w121:errorcluster)  [unwired: 13 in]
          n171 = call <vilib>:"DAQmx Clear Task.vi"("task in"=w126, "error in"=w127) -> ("error out"=w120:errorcluster)  [unwired: 13 in]
          n172 = Merge Errors(w121, w120, w112, w111) -> (w119:errorcluster)
        }
      }
      n173 = Unbundle(w6) -> ("Boolean"=w78:bool, "VISA out"=w77:refnum<visa-resource-name>, "error out"=w15:errorcluster)
      n174 = call-poly <vilib>:"Write To Spreadsheet File.vi"("append to file? (new file:F)"=TRUE, "2D data"=w62, "file path (dialog if empty)"=w71) -> ()  [unwired: 5 in, 1 out]
      n175 = Unbundle(w8) -> (w81:bool, "VISA resource name out"=w80:refnum<visa-resource-name>, "error out"=w79:errorcluster)
      n176 = Unbundle(w7) -> (w18:bool, "VISA resource name out"=w17:refnum<visa-resource-name>, "error out"=w16:errorcluster)
      n177 = Unbundle(w10) -> (w67:bool, "VISA resource name out"=w66:refnum<visa-resource-name>, "error out"=w65:errorcluster)
      n178 = call "arduino_close_subIV 11-08-2017.vi"("arduino addresses out"=w11) -> ()  [unwired: 11 in]
      n179 = Unbundle(w9) -> ("Boolean"=w75:bool, "VISA resource name out"=w74:refnum<visa-resource-name>, "error out"=w73:errorcluster)
      n180 = case shown="False" w78 {
        tunnel: [w201 w204] -> w14
        tunnel: w77 -> [_ w203]
        tunnel: w15 -> [w201 w202]
        frame False {
          # "SRS-200 close"
        }
        frame True {
          # "SRS-200 close"
          n181 = call "srsQcm200Close.vi"("error in"=w202, "Visa in"=w203) -> ("error out"=w204:errorcluster)  [unwired: 3 in]
        }
      }
      n182 = case shown="True" w18 {
        tunnel: w17 -> [_ w92]
        tunnel: w16 -> [w89 w91]
        tunnel: [w89 w90] -> w59
        frame False {
          # "Keithley-2100 close"
        }
        frame True {
          # "Keithley-2100 close"
          n183 = call "Close.vi"("VISA resource name"=w92, "error in (no error)"=w91) -> ("error out"=w90:errorcluster)  [unwired: 17 in]
        }
      }
      n184 = case shown="True" w81 {
        tunnel: w80 -> [_ w220]
        tunnel: w79 -> [w217 w219]
        tunnel: [w217 w218] -> w82
        frame False {
          # "Keithley-2420 close"
        }
        frame True {
          # "Keithley-2420 close"
          n185 = call "Enable Output.vi"("error in (no error)"=w219, "Enable Output (T: Enable)"=FALSE, "VISA resource name"=w220) -> ("error out"=w221:errorcluster, "VISA resource name out"=w223:refnum<visa-resource-name>)  [unwired: 7 in]
          n186 = call "Close.vi"("error in (no error)"=w221, "VISA resource name"=w223) -> ("error out"=w218:errorcluster)  [unwired: 9 in]
        }
      }
      n187 = case shown="True" w67 {
        tunnel: w66 -> [_ w158]
        tunnel: w65 -> [w156 w157]
        tunnel: [w156 w159] -> w64
        frame False {
          # "Keithley-6430 close"
        }
        frame True {
          # "Keithley-6430 close"
          n188 = call "Enable Output.vi"("error in (no error)"=w157, "Enable Output (F:Off)"=FALSE ("Output (F:Off)"), "VISA resource name"=w158) -> ("error out"=w160:errorcluster, "VISA resource name out"=w161:refnum<visa-resource-name>)  [unwired: 7 out]
          n189 = call "Close.vi"("error in (no error)"=w160, "VISA resource name"=w161) -> ("error out"=w159:errorcluster)  [unwired: 9 out]
        }
      }
      n190 = case shown="True" w75 {
        tunnel: w74 -> [_ w189]
        tunnel: w73 -> [w186 w188]
        tunnel: [w186 w187] -> w72
        frame False {
          # "J-KEM close"
        }
        frame True {
          # "J-KEM close"
          n191 = VISA Close(VISA resource name=w189, error in (no error)=w188) -> (error out=w187:errorcluster)
        }
      }
      n192 = call <vilib>:"Simple Error Handler.vi"("error in (no error)"=w56) -> ()  [unwired: 4 in, 5 out]
      n193 = flat-sequence {
        tunnel: w14 -> [w88]
        tunnel: [w88] -> w13
        frame #0 {
          w87 = FALSE ("saving data?")
          # "re-initialize settings"
          n194 = property on="saving data?" class="Bool (strict)"("Value"=w87) -> ()  [unwired: 2 in, 2 out]
          n195 = property on="Run Sequence" class="Bool (strict)"("Value"=w87) -> ()  [unwired: 2 in, 2 out]
        }
      }
      n196 = Merge Errors(w64, w72, w82, w59, w13) -> (w83:errorcluster)
      n197 = call <vilib>:"Simple Error Handler.vi"("error in (no error)"=w83) -> ()  [unwired: 4 in, 5 out]
    }
  }
